vi "Add Pointer at Index.vi"(4 "Insertion Index":i32=-1, 6 "Unique ID":string, 11 "Linked List Definition in":refnum<class "Linked List Definition.lvclass">) -> (3 "Linked List Definition out":refnum<class "Linked List Definition.lvclass">)   [LabVIEW 2020, in "Linked Lists.lvlib" / "Linked List Definition.lvclass"]
uses:
  <vilib>/gpm_packages/@cs/linked-list/Source/Linked List/Linked List Definition/Linked List Definition.lvclass
  <vilib>/gpm_packages/@cs/linked-list/Source/Linked List/Linked List Definition/Linked List Definition.lvclass/Linked List Definition.ctl
panel:
  in  "Pointer ID":string
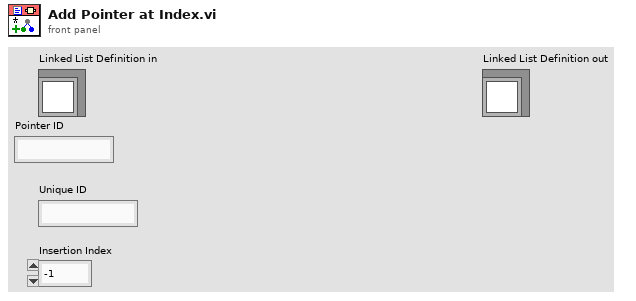
[diagram p1: front panel]
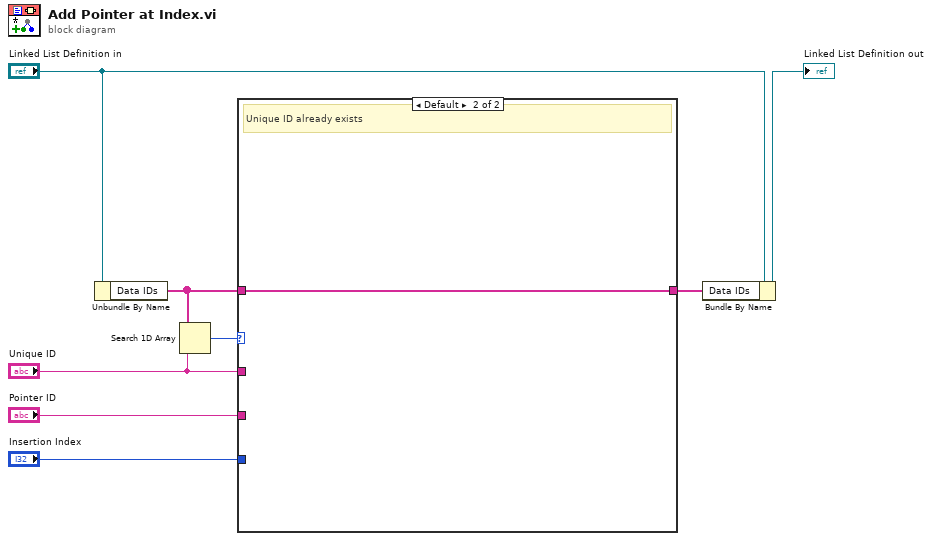
[diagram p0: block diagram]
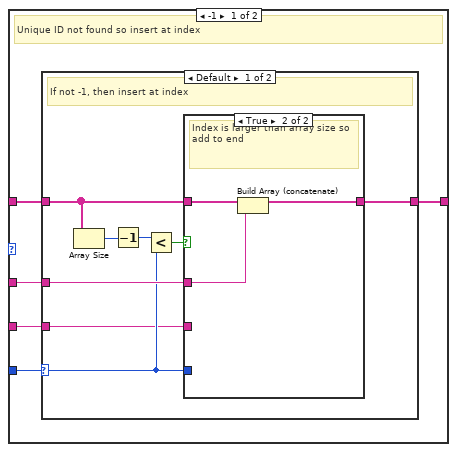
[diagram p2: hidden frame]
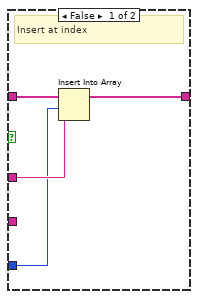
[diagram p3: hidden frame]
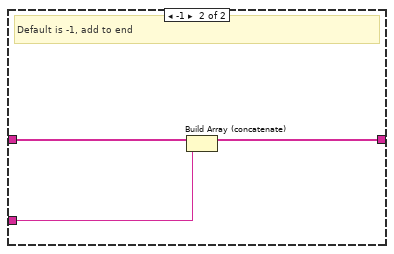
[diagram p4: hidden frame]
diagram:
  n1 = Unbundle By Name("Linked List Definition in") -> ("Data IDs"=w7:string[])
  n2 = Search 1D Array(1D array=w7, element="Unique ID") -> (index of element=w8:i32)  [unwired: 1 in]
  n3 = case shown="Default" w8 {
    tunnel: w7 -> [w13 w32]
    tunnel: "Unique ID" -> [w12 _]
    tunnel: [w11 w32] -> w2
    tunnel: "Insertion Index" -> [w10 _]
    tunnel: "Pointer ID" -> [w9 _]
    frame -1 {
      # "Unique ID not found so insert at index"
      n4 = case shown="Default" w10 {
        selector: w10 -> [w16 _]
        tunnel: w13 -> [w17 w31]
        tunnel: w12 -> [w20 w30]
        tunnel: [w21 w29] -> w11
        tunnel: w9 -> [w14 _]
        frame Default {
          # "If not -1, then insert at index"
          n5 = Array Size(array=w17) -> (size(s)=w19:i32)
          n6 = Decrement(x=w19) -> (x-1=w18:i32)
          n7 = Less?(x=w18, y=w16) -> (x < y?=w15:bool)
          n8 = case shown="True" w15 {
            tunnel: [w25 w27] -> w21
            tunnel: w20 -> [w24 w26]
            tunnel: w17 -> [w23 w28]
            tunnel: w16 -> [w22 _]
            tunnel: w14 -> [_ _]
            frame False {
              # "Insert at index"
              n9 = Insert Into Array(array=w23, index=w22, new element=w24) -> (w25:string[])
            }
            frame True {
              # "Index is larger than array size so add to end"
              n10 = Build Array (concatenate)(w28, w26) -> (w27:string[])
            }
          }
        }
        frame -1 {
          # "Default is -1, add to end"
          n11 = Build Array (concatenate)(w31, w30) -> (w29:string[])
        }
      }
    }
    frame Default {
      # "Unique ID already exists"
    }
  }
  n12 = Bundle By Name(cluster="Linked List Definition in", "Data IDs"=w2) -> (→"Linked List Definition out":refnum<class "Linked List Definition.lvclass">)
